vi "CurrentWebServiceStatus.vi"(8 "New WebService Status":T1, 11 "Operation":T2) -> (3 "Current WebService Status":T1)   [LabVIEW 2024]
uses:
  DataTypes/WebServiceStatus.ctl
  DataTypes/OperationTypeForFunctionalGlobalVariable.ctl
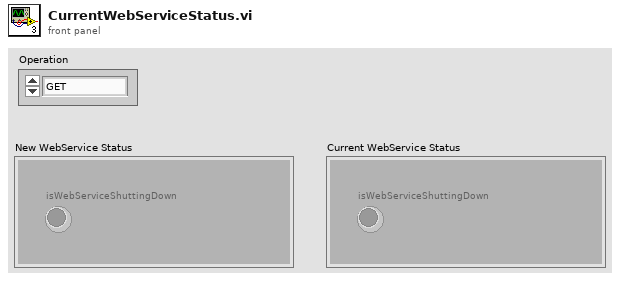
[diagram p1: front panel]
types:
  T1 = typedef "WebServiceStatus.ctl" = cluster{"isWebServiceShuttingDown":bool}
  T2 = typedef "OperationTypeForFunctionalGlobalVariable.ctl" = enum16{"GET", "SET"}
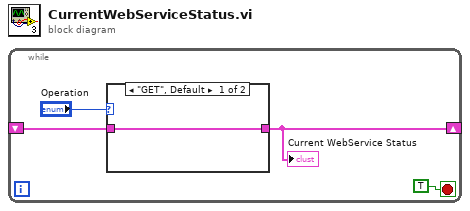
[diagram p0: block diagram]
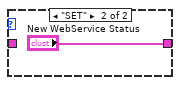
[diagram p2: hidden frame]
diagram:
  n1 = while {
    shift-right: [w1] -> _
    shift-left: _ -> [w3]
    stop <- TRUE stop-if-true
    n2 = case shown="\"GET\", Default" "Operation" {
      tunnel: w3 -> [w5 _]
      tunnel: [w5 "New WebService Status"] -> w1
      frame "GET", Default {
      }
      frame "SET" {
      }
    }
    "Current WebService Status" <- w1
  }
